vi "Keithley2420_IV.vi"() -> ()   [LabVIEW 2014]
uses:
  Environmental Chamber LabVIEW and Instruments/Drivers and Software/keithley_6430/Keithley 6430/Public/Data/Read (Single Point).vi
  Environmental Chamber LabVIEW and Instruments/Drivers and Software/LabVIEW 8.2 Drivers/keithley_24xx/Keithley 24XX/Public/Data/Read (Single Point).vi
  <vilib>/Utility/file.llb/Write To Spreadsheet File (string).vi
  Environmental Chamber LabVIEW and Instruments/Drivers and Software/keithley_24xx/Keithley 24XX/Keithley 24XX.lvlib
  Environmental Chamber LabVIEW and Instruments/Drivers and Software/keithley_6430/Keithley 6430/Keithley 6430.lvlib
panel:
  out "appended array":sgl[][](array[numeric])
  in  "Tab Control":enum32{"2420", "6430"}(tab)
  out "V":dbl
  out "XY Graph":cluster{"Y":dbl[], "Y":dbl[]}[](graph)
  out "I":sgl
  in  "STOP":bool
  out "Resistance":sgl
  out "Waveform Chart":sgl(graph)
  out "I 2":sgl
  out "6430":cluster{"Y":dbl[], "Y":dbl[]}[](graph)
  out "V 2":dbl
  in  "STOP 3":bool
  in  "Instrument":u16(ring)=1 items=["Keithley 6430", "Keithley 2420"]
  in  "File notes":string="50% RH"
  in  "# of steps":dbl=30.0
  in  "Vf":dbl=0.3
  in  "Vi":dbl
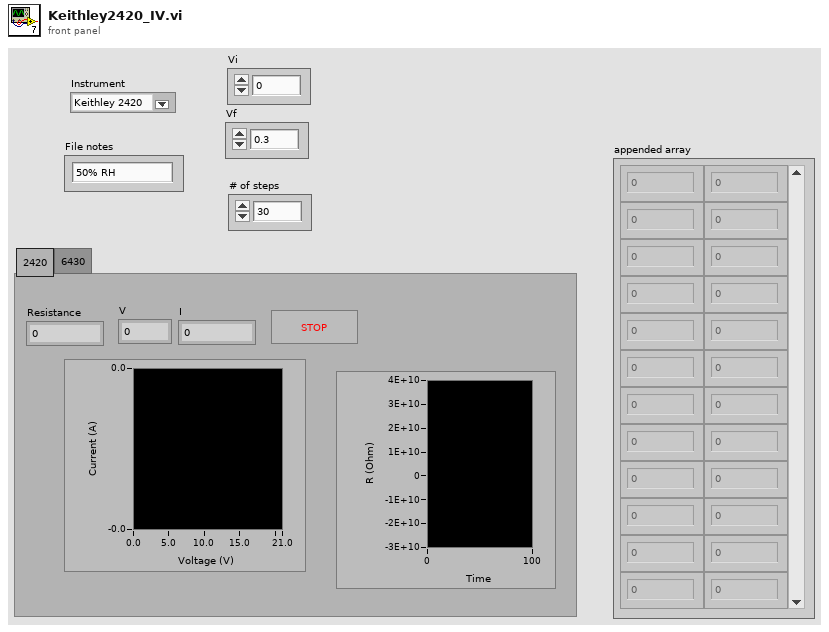
[diagram p1: front panel]
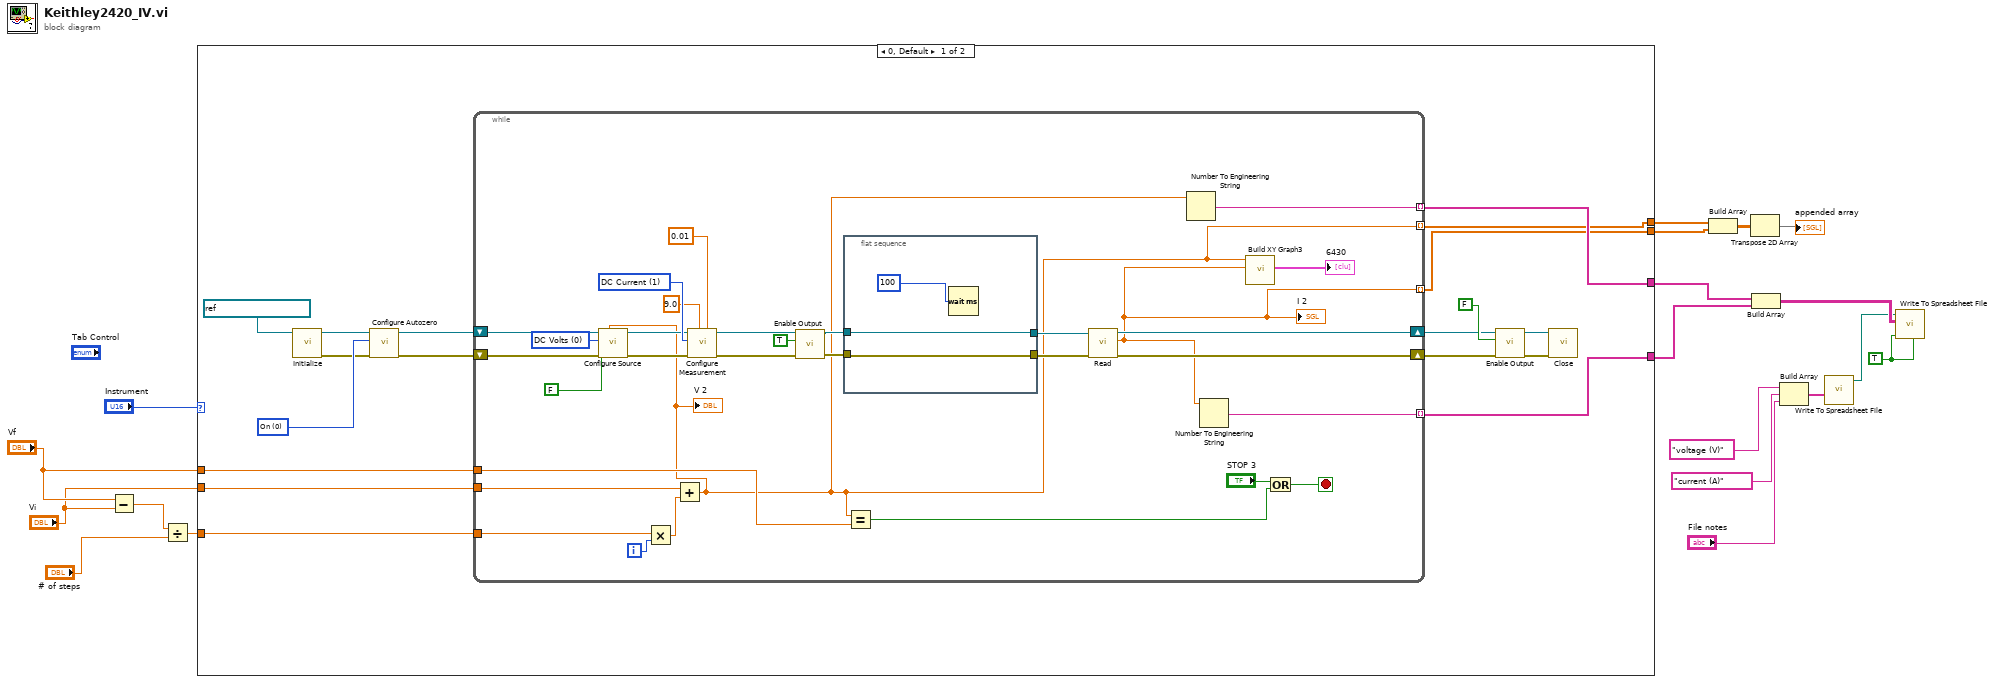
[diagram p0: block diagram]
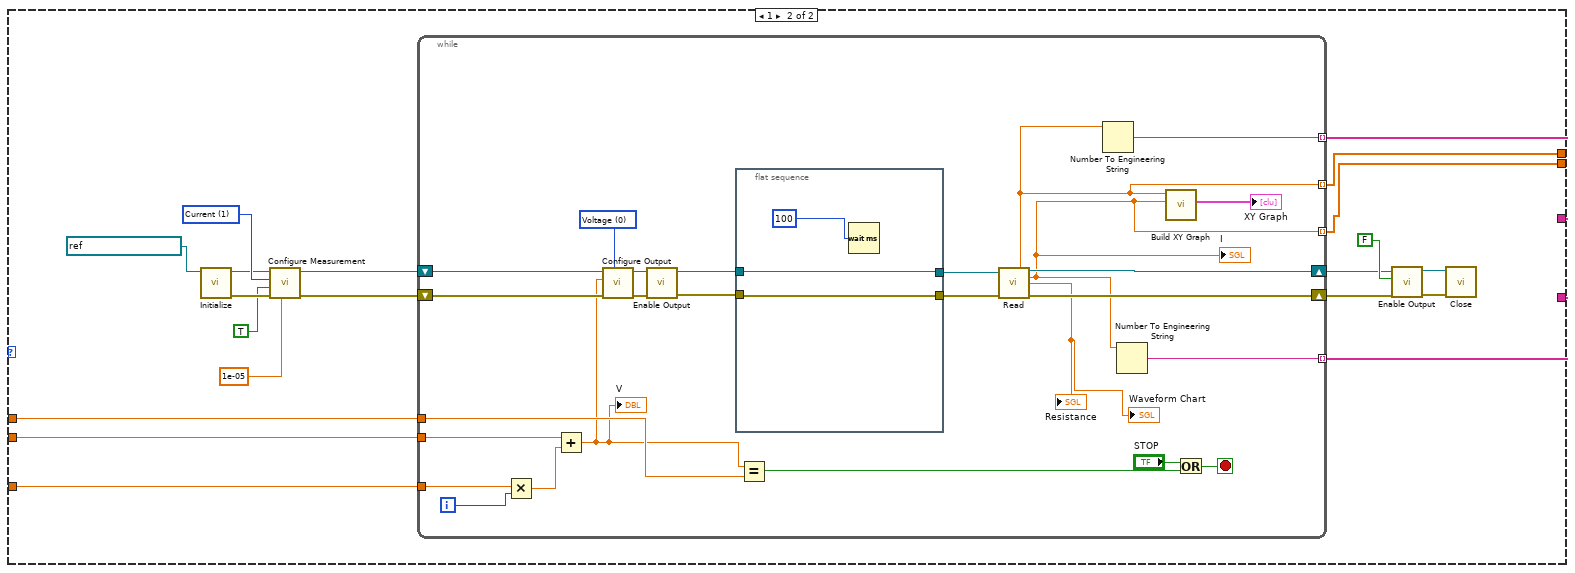
[diagram p2: hidden frame]
diagram:
  w13 = TRUE ("transpose? (no:F)")
  n1 = Subtract(x="Vf", y="Vi") -> (x-y=w18:dbl)
  n2 = Divide(x=w18, y="# of steps") -> (x/y=w14:dbl)
  n3 = case shown="0, Default" "Instrument" {
    tunnel: "Vf" -> [w37 w80]
    tunnel: "Vi" -> [w36 w79]
    tunnel: w14 -> [w35 w78]
    tunnel: [w34 w77] -> w6
    tunnel: [w33 w76] -> w5
    tunnel: [w21 w73] -> w2
    tunnel: [w20 w72] -> w1
    frame 0, Default {
      w30 = u16 0 items=["On", "Off", "Once"] ("Autozero  (0: On)")
      n4 = call "Initialize.vi"("VISA resource name"=refnum<visa-resource-name> "GPIB0::29::INSTR") -> ("error out"=w29:errorcluster, "VISA resource name out"=w31:refnum<visa-resource-name>)  [unwired: 7 in, 2 out]
      n5 = call "Configure Autozero.vi"("error in (no error)"=w29, "Autozero  (0: On)"=w30, "VISA resource name"=w31) -> ("error out"=w27:errorcluster, "VISA resource name out"=w28:refnum<visa-resource-name>)  [unwired: 7 in]
      n6 = while {
        tunnel: [w68] -> w33 mode=indexing
        shift-right: [w53] -> w23
        shift-left: w27 -> [w47]
        shift-right: [w52] -> w22
        shift-left: w28 -> [w48]
        tunnel: w35 -> [w67]
        tunnel: w36 -> [w66]
        tunnel: [w65] -> w34 mode=indexing
        tunnel: w37 -> [w64]
        tunnel: [w43] -> w21 mode=indexing
        tunnel: [w42] -> w20 mode=indexing
        i -> [w59]
        stop <- w62 stop-if-true
        w49 = u16 1 items=["DC Volts", "DC Current"] ("Measure Function (1: DC Current)")
        w50 = u16 0 items=["DC Volts", "DC Current"] ("Source Function (0: DC Volts)")
        n7 = Multiply(x=w67, y=w59) -> (x*y=w60:dbl)
        n8 = Add(x=w66, y=w60) -> (x+y=w43:dbl)
        "V 2" <- w43
        n9 = call "Configure Source.vi"("V-Source Level [V]"=w43, "error in (no error)"=w47, "Auto Range (T:Enable)"=FALSE, "Source Function (0: DC Volts)"=w50, "VISA resource name"=w48) -> ("error out"=w51:errorcluster, "VISA resource name out"=w46:refnum<visa-resource-name>)  [unwired: 5 in]
        n10 = call "Configure Measurement.vi"("Current Compliance [A]"=0.01, "Voltage Compliance [V]"=9.0, "error in (no error)"=w51, "Measure Function (1: DC Current)"=w49, "VISA resource name"=w46) -> ("error out"=w44:errorcluster, "VISA resource name out"=w45:refnum<visa-resource-name>)  [unwired: 5 in]
        n11 = call "Enable Output.vi"("error in (no error)"=w44, "Enable Output (F:Off)"=TRUE, "VISA resource name"=w45) -> ("error out"=w56:errorcluster, "VISA resource name out"=w57:refnum<visa-resource-name>)  [unwired: 7 in]
        n12 = flat-sequence {
          tunnel: [w71] -> w55
          tunnel: w57 -> [w71]
          tunnel: w56 -> [w70]
          tunnel: [w70] -> w54
          frame #0 {
            n13 = Wait (ms)(milliseconds to wait=u32 100) -> ()  [unwired: 1 out]
          }
        }
        n14 = Equal?(x=w43, y=w64) -> (x = y?=w63:bool)
        n15 = call-poly "Read.vi"("error in (no error)"=w54, "VISA resource name"=w55) -> ("error out"=w53:errorcluster, "Measurement"=w42:dbl, "VISA resource name out"=w52:refnum<visa-resource-name>)  [unwired: 7 in]
        "I 2" <- w42
        n16 = Number To Engineering String(4:w43) -> (0:w65:string)  [unwired: 3 in]
        n17 = Number To Engineering String(4:w42) -> (0:w68:string)  [unwired: 3 in]
        n18 = call "Build XY Graph3"("Y Input"=w42, "X Input"=w43) -> ("XY Graph"=→"6430":cluster{"X":dbl[], "Y":dbl[]}[])  [unwired: 8 in, 1 out]
        n19 = Or(x="STOP 3", y=w63) -> (x .or. y?=w62:bool)
      }
      n20 = call "Enable Output.vi"("error in (no error)"=w23, "Enable Output (F:Off)"=FALSE ("Enable Output (T: Enable)"), "VISA resource name"=w22) -> ("error out"=w24:errorcluster, "VISA resource name out"=w25:refnum<visa-resource-name>)  [unwired: 7 in]
      n21 = call "Close.vi"("error in (no error)"=w24, "VISA resource name"=w25) -> ()  [unwired: 9 in, 1 out]
    }
    frame 1 {
      w85 = u16 1 items=["Volts", "Current", "Resistance"] ("Function (0: Volts)")
      n22 = call "Initialize.vi"("VISA resource name"=refnum<visa-resource-name> "GPIB1::24::INSTR") -> ("error out"=w81:errorcluster, "VISA resource name out"=w82:refnum<visa-resource-name>)  [unwired: 9 in]
      n23 = call "Configure Measurement.vi"("Manual Range (1.0)"=1e-05, "error in (no error)"=w81, "Enable Auto Range (T:Enable)"=TRUE, "Function (0: Volts)"=w85, "VISA resource name"=w82) -> ("error out"=w84:errorcluster, "VISA resource name out"=w83:refnum<visa-resource-name>)  [unwired: 5 in]
      n24 = while {
        tunnel: [w110] -> w76 mode=indexing
        shift-right: [w116] -> w87
        shift-left: w84 -> [w115]
        shift-right: [w117] -> w88
        shift-left: w83 -> [w114]
        tunnel: w78 -> [w105]
        tunnel: w79 -> [w104]
        tunnel: [w103] -> w77 mode=indexing
        tunnel: w80 -> [w102]
        tunnel: [w93] -> w73 mode=indexing
        tunnel: [w92] -> w72 mode=indexing
        i -> [w96]
        stop <- w100 stop-if-true
        w111 = u16 0 items=["Voltage", "Current"] ("Source Mode  (0: Voltage)")
        n25 = Multiply(x=w105, y=w96) -> (x*y=w97:dbl)
        n26 = Add(x=w104, y=w97) -> (x+y=w98:dbl)
        "V" <- w98
        n27 = call "Configure Output.vi"("Source Mode  (0: Voltage)"=w111, "error in (no error)"=w115, "Output Level (0)"=w98, "VISA resource name"=w114) -> ("error out"=w113:errorcluster, "VISA resource name out"=w112:refnum<visa-resource-name>)  [unwired: 6 in]
        n28 = call "Enable Output.vi"("error in (no error)"=w113, "VISA resource name"=w112) -> ("error out"=w106:errorcluster, "VISA resource name out"=w109:refnum<visa-resource-name>)  [unwired: 8 in]
        n29 = flat-sequence {
          tunnel: [w120] -> w108
          tunnel: w109 -> [w120]
          tunnel: w106 -> [w119]
          tunnel: [w119] -> w107
          frame #0 {
            n30 = Wait (ms)(milliseconds to wait=u32 100) -> ()  [unwired: 1 out]
          }
        }
        n31 = Equal?(x=w98, y=w102) -> (x = y?=w101:bool)
        n32 = call-poly "Read.vi"("VISA resource name"=w108, "error in (no error)"=w107) -> ("Voltage"=w93:sgl, "VISA resource name out"=w117:refnum<visa-resource-name>, "Current"=w92:sgl, "Resistance"=→"Resistance" →"Waveform Chart":sgl, "error out"=w116:errorcluster)  [unwired: 7 in, 2 out]
        "I" <- w92
        n33 = Number To Engineering String(4:w93) -> (0:w103:string)  [unwired: 3 in]
        n34 = Number To Engineering String(4:w92) -> (0:w110:string)  [unwired: 3 in]
        n35 = call "Build XY Graph"("Y Input"=w92, "X Input"=w93) -> ("XY Graph"=→"XY Graph":cluster{"X":dbl[], "Y":dbl[]}[])  [unwired: 8 in, 1 out]
        n36 = Or(x="STOP", y=w101) -> (x .or. y?=w100:bool)
      }
      n37 = call "Enable Output.vi"("error in (no error)"=w87, "Enable Output (T: Enable)"=FALSE, "VISA resource name"=w88) -> ("error out"=w89:errorcluster, "VISA resource name out"=w91:refnum<visa-resource-name>)  [unwired: 7 in]
      n38 = call "Close.vi"("error in (no error)"=w89, "VISA resource name"=w91) -> ()  [unwired: 9 in, 1 out]
    }
  }
  n39 = Build Array(w2, w1) -> (w3:dbl[][])
  n40 = Transpose 2D Array(2D array=w3) -> (transposed array=→"appended array":dbl[][])
  n41 = Build Array(w6, w5) -> (w12:string[][])
  n42 = Build Array("voltage (V)", "current (A)", "File notes") -> (w10:string[])
  n43 = call-poly <vilib>:"Write To Spreadsheet File.vi"("1D data"=w10) -> ("new file path (Not A Path if cancelled)"=w9:path)  [unwired: 7 in]
  n44 = call-poly <vilib>:"Write To Spreadsheet File.vi"("transpose? (no:F)"=w13, "append to file? (new file:F)"=w13, "2D data"=w12, "file path (dialog if empty)"=w9) -> ()  [unwired: 4 in, 1 out]
